vi "Device Parameters to Configuration Elements.vi"(11 "device parameters":T1) -> (0 "core number":i32, 1 "number":i32, 2 "number caption":string, 3 "initialization method":T2)   [LabVIEW 2020, in "Ballard MIL-STD-1553 System Explorer.lvlib" / "Implementation.lvlib"]
uses:
  Implementation.lvlib
  Scripting/Constants.vi
  Scripting/Ballard MIL-STD-1553 Scripting.lvlib
  Shared/Initialization Method.ctl
  Shared/Device Parameters.ctl
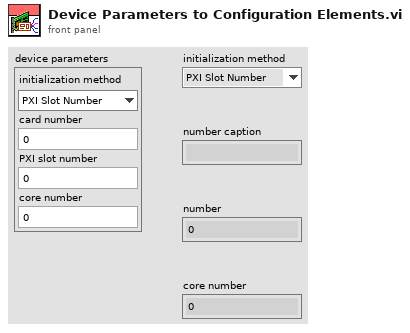
[diagram p1: front panel]
types:
  T1 = typedef "Device Parameters.ctl" = cluster{"initialization method":T2, "card number":i32, "PXI slot number":i32, "core number":i32}
  T2 = typedef "Initialization Method.ctl" = enum16{"PXI Slot Number", "Card Number"}
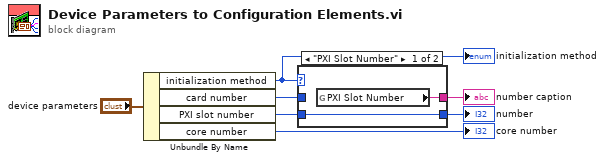
[diagram p0: block diagram]
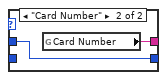
[diagram p2: hidden frame]
diagram:
  n1 = Unbundle By Name("device parameters") -> ("initialization method"=w7:T2, "card number"=w3:i32, "PXI slot number"=w4:i32, "core number"=→"core number":i32)
  "initialization method" <- w7
  n2 = case shown="\"PXI Slot Number\"" w7 {
    tunnel: w3 -> [_ w11]
    tunnel: w4 -> [w8 _]
    tunnel: [w8 w11] -> w5
    tunnel: [w9 w10] -> w6
    frame "PXI Slot Number" {
      n3 = global read "Constants.vi" "PXI Slot Number"() -> (w9:string)
    }
    frame "Card Number" {
      n4 = global read "Constants.vi" "Card Number"() -> (w10:string)
    }
  }
  "number caption" <- w6
  "number" <- w5
